vi "Configure Current.vi"(4 "Switch Mode (0: Continuous)":i32(ring) items=["Continuous", "Fast"], 6 "Current Integration Time (10: 10)":dbl(ring)=10.0 items=["0.02"=0.02, "0.2"=0.2, "1"=1.0, "10"=10.0, "100"=100.0], 7 "Terminal Type (3: 3 A Terminal)":i32(ring)=3 items=["3 A Terminal"=3, "10 A Terminal"=10], 8 "error in (no error)":errorcluster, 9 "Current Type (0: AC)":i32(ring) items=["AC", "DC"], 10 "Current Bandwidth (20 Hz)":dbl(ring)=20.0 items=["3"=3.0, "20"=20.0, "200"=200.0], 11 "VISA resource name":refnum<visa-resource-name>) -> (0 "error out":errorcluster, 3 "VISA resource name out":refnum<visa-resource-name>)   [LabVIEW 2013, in "Agilent 3446X Series.lvlib"]
doc: "Configures current settings.\n\n<b>Note(s):</b>\nThis vi is not supported for EDU34450A model."
uses:
  <instrlib>/Agilent 3446X Series/Agilent 3446X Series.lvlib
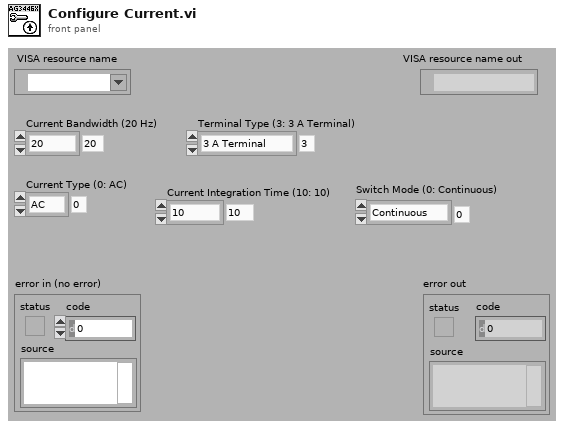
[diagram p1: front panel]
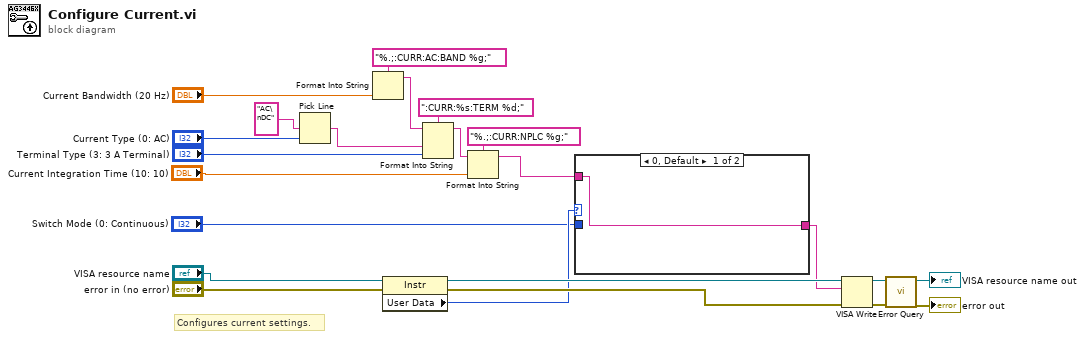
[diagram p0: block diagram]
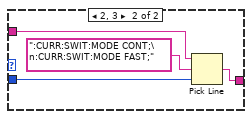
[diagram p2: hidden frame]
diagram:
  # "Configures current settings."
  n1 = Pick Line(multi-line string="AC\nDC", line index="Current Type (0: AC)") -> (output string=w12:string)  [unwired: 1 out]
  n2 = Format Into String(format string="%.;:CURR:AC:BAND %g;", "Current Bandwidth (20 Hz)") -> (resulting string=w19:string)  [unwired: 2 in, 1 out]
  n3 = property class="Instr"(reference="VISA resource name", error in="error in (no error)") -> (reference out=w10:refnum<visa-resource-name>, error out=w9:errorcluster, "User Data"=w7:u32)
  n4 = Format Into String(format string=":CURR:%s:TERM %d;", initial string=w19, w12, "Terminal Type (3: 3 A Terminal)") -> (resulting string=w2:string)  [unwired: 1 in, 1 out]
  n5 = Format Into String(format string="%.;:CURR:NPLC %g;", initial string=w2, "Current Integration Time (10: 10)") -> (resulting string=w1:string)  [unwired: 1 in, 1 out]
  n6 = case shown="0, Default" w7 {
    tunnel: [w24 w25] -> w5
    tunnel: "Switch Mode (0: Continuous)" -> [_ w27]
    tunnel: w1 -> [w24 w26]
    frame 0, Default {
    }
    frame 2, 3 {
      n7 = Pick Line(string ("")=w26, multi-line string=":CURR:SWIT:MODE CONT;\n:CURR:SWIT:MODE FAST;", line index=w27) -> (output string=w25:string)
    }
  }
  n8 = VISA Write(VISA resource name=w10, write buffer=w5, error in (no error)=w9) -> (VISA resource name out=w16:refnum<visa-resource-name>, error out=w15:errorcluster)  [unwired: 1 out]
  n9 = call <instrlib>:"Error Query.vi"("error in (no error)"=w15, "VISA resource name"=w16) -> ("error out"=→"error out":errorcluster, "VISA resource name out"=→"VISA resource name out":refnum<visa-resource-name>)  [unwired: 8 out]
